vi "SetSyncNotifier.vi"(8 "error in (no error)":errorcluster, 10 "Sync Notifier":refnum<notifier>, 11 "SMO in":refnum<class "SMO.lvclass">) -> (0 "error out":errorcluster, 3 "SMO out":refnum<class "SMO.lvclass">)   [LabVIEW 2013, in "SMO.lvclass"]
uses:
  SMO.lvclass
  SMO.lvclass/SMO.ctl
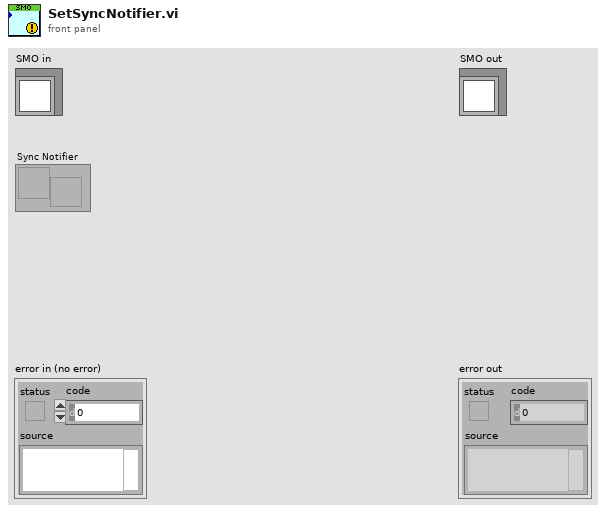
[diagram p1: front panel]
types:
  T1 = typedef "SMO.lvclass/PrivateData--Ref.ctl" = refnum<data-value>
  T2 = typedef "SMO.lvclass/PrivateData--Cluster.ctl" = cluster{"Parent Call":T3, "Registered Processes":T4[], "Sync Notifier":refnum<notifier>, "Process Error Notifier":refnum<notifier>, "Protected Events":T5, "Public Events":T6, "SMO State":T7, "[Dependencies]":T8[], "[Attributes]":refnum<class "Attribute.lvclass">[], "Launcher Close":refnum<notifier>}
  T3 = typedef "SMO.lvclass/Parent Call--Enum.ctl" = enum16{"Allows parent to run", "Does not request parent to run"}
  T4 = typedef "SMO.lvclass/RegisteredProcessData--Cluster.ctl" = cluster{"Name":string, "Static VI Ref":refnum<vi>, "Running":bool, "NotifierRef":u32}
  T5 = typedef "SMO.lvclass/Protected Events.ctl" = cluster{"StopProcesses":refnum<user-event>, "AbortProcesses":refnum<user-event>, "Config Changed":refnum<user-event>}
  T6 = typedef "SMO.lvclass/Public Events.ctl" = cluster{"Error":refnum<user-event>, "State":refnum<user-event>}
  T7 = typedef "SMO.lvclass/SMOState --Enum.ctl" = enum16{"unknown", "Created", "Started", "Stopped"}
  T8 = typedef "SMO.lvclass/SMO Dependency--Cluster.ctl" = cluster{"Dependency":refnum<class "SMO.lvclass">, "Level":string}
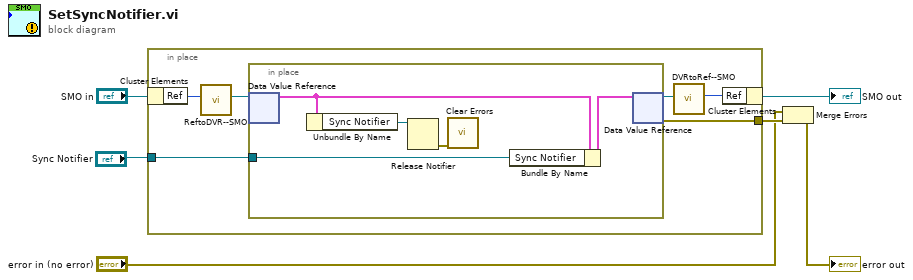
[diagram p0: block diagram]
diagram:
  n1 = in-place {
    in-place-border: [w9] -> w4
    in-place-border: "Sync Notifier" -> [w8]
    n2 = in-place-cluster #1("SMO in") -> ("Ref"=w12:u32)
    n3 = call "ReftoDVR--SMO.vi"("Ref"=w12) -> ("Ref"=w10:T1)  [unwired: 10 in]
    n4 = in-place {
      in-place-border: w8 -> [w17]
      n5 = in-place-dvr #2(w10) -> (w15:T2)  [unwired: 1 out]
      n6 = Unbundle By Name(w15) -> ("Sync Notifier"=w14:refnum<notifier>)
      n7 = Release Notifier(notifier=w14) -> (error out=w13:errorcluster)  [unwired: 2 in, 2 out]
      n8 = call <vilib>:"Clear Errors.vi"("error in (no error)"=w13) -> ()  [unwired: 6 in, 1 out]
      n9 = Bundle By Name(cluster=w15, "Sync Notifier"=w17) -> (w16:T2)
      n10 = in-place-dvr #2(w16) -> (w7:T1, w9:errorcluster)
    }
    n11 = call "DVRtoRef--SMO.vi"("Ref"=w7) -> ("Ref"=w11:u32)  [unwired: 10 in]
    n12 = in-place-cluster #1("Ref"=w11) -> (→"SMO out":refnum<class "SMO.lvclass">)
  }
  n13 = Merge Errors("error in (no error)", w4) -> (→"error out":errorcluster)
